vi "3.5.vi"() -> ()   [LabVIEW 2019]
panel:
  out "Waveform Graph":dbl[](graph)
  in  "kinetic friction":dbl
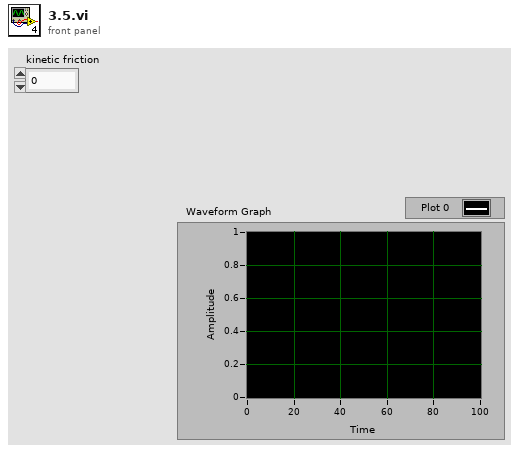
[diagram p1: front panel]
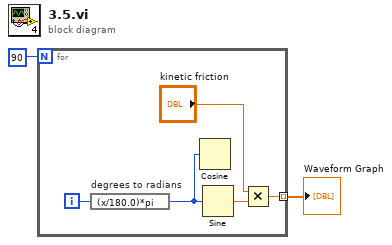
[diagram p0: block diagram]
diagram:
  n1 = for {
    N: 90 -> [_]
    tunnel: [w3] -> w1 mode=indexing
    i -> [w7]
    n2 = expression code="(x/180.0)*pi" "degrees to radians"(w7) -> (w6:i32)
    n3 = Cosine(x=w6) -> ()  [unwired: 1 out]
    n4 = Sine(x=w6) -> (sin(x)=w5:dbl)
    n5 = Multiply(x="kinetic friction", y=w5) -> (x*y=w3:dbl)
  }
  "Waveform Graph" <- w1
